vi "AutonSelector.vi"(10 "Buttons1":T1, 11 "Buttons in":T1) -> (0 "Current Auton":dbl, 1 "sorted array":string[](array[string]), 2 "Auton Array":dbl[][](array[numeric]), 3 "Number of Auton Files":dbl)   [LabVIEW 2013]
uses:
  <vilib>/Rock Robotics/WPI/Joystick/WPI_JoystickButtonState.ctl
  Robot Global Data.vi
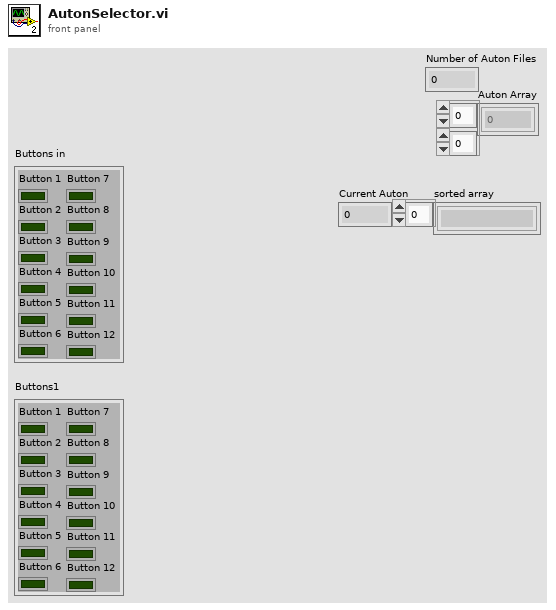
[diagram p1: front panel]
types:
  T1 = typedef "WPI_JoystickButtonState.ctl" = cluster{"Button 1":bool, "Button 2":bool, "Button 3":bool, "Button 4":bool, "Button 5":bool, "Button 6":bool, "Button 7":bool, "Button 8":bool, "Button 9":bool, "Button 10":bool, "Button 11":bool, "Button 12":bool}
  T2 = cluster{"Setpoint 1":dbl, "Setpoint 2":dbl, "Setpoint 3":dbl, "Setpoint 4":dbl, "RotLow":dbl, "RotHigh":dbl, "ExtLow":dbl, "ExtHigh":dbl}
  T3 = cluster{"FlipperLeftUp":dbl, "FlipperLeftDown":dbl, "FlipperRightUp":dbl, "FlipperRightDown":dbl, "KickerLeftBack":dbl, "KickerLeftForward":dbl, "KickerRightBack":dbl, "KickerRightForward":dbl}
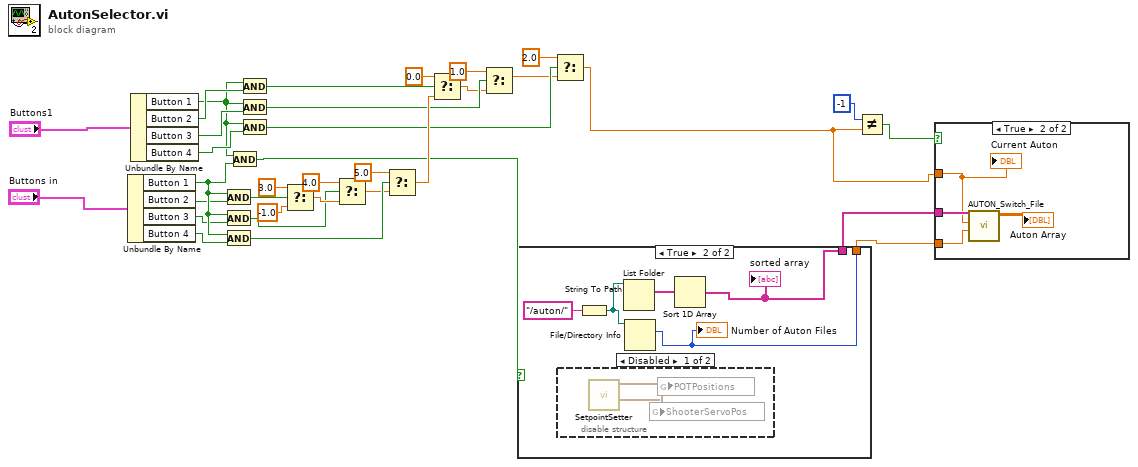
[diagram p0: block diagram]
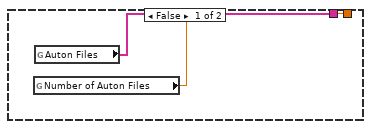
[diagram p3: hidden frame]
diagram:
  n1 = Unbundle By Name("Buttons in") -> ("Button 1"=w6:bool, "Button 2"=w4:bool, "Button 3"=w5:bool, "Button 4"=w7:bool)
  n2 = Unbundle By Name("Buttons1") -> ("Button 1"=w25:bool, "Button 2"=w26:bool, "Button 3"=w27:bool, "Button 4"=w28:bool)
  n3 = And(x=w6, y=w4) -> (x .and. y?=w8:bool)
  n4 = And(x=w6, y=w5) -> (x .and. y?=w11:bool)
  n5 = And(x=w6, y=w7) -> (x .and. y?=w17:bool)
  n6 = And(x=w25, y=w6) -> (x .and. y?=w15:bool)
  n7 = And(x=w25, y=w26) -> (x .and. y?=w24:bool)
  n8 = And(x=w25, y=w27) -> (x .and. y?=w22:bool)
  n9 = And(x=w25, y=w28) -> (x .and. y?=w29:bool)
  n10 = Select(t=3.0, s=w8, f=-1.0) -> (s? t:f=w12:dbl)
  n11 = Select(t=4.0, s=w11, f=w12) -> (s? t:f=w14:dbl)
  n12 = Select(t=5.0, s=w17, f=w14) -> (s? t:f=w30:dbl)
  n13 = Select(t=0.0, s=w24, f=w30) -> (s? t:f=w21:dbl)
  n14 = Select(t=1.0, s=w22, f=w21) -> (s? t:f=w19:dbl)
  n15 = case shown="True" w15 {
    tunnel: [w35 w37] -> w1
    tunnel: [w36 w38] -> w3
    frame False {
      n16 = global read "Robot Global Data.vi" "Number of Auton Files"() -> (w35:dbl)
      n17 = global read "Robot Global Data.vi" "Auton Files"() -> (w36:string[])
    }
    frame True {
      n18 = disable-structure shown="Disabled" {
        frame Disabled {
          n19 = call "SetpointSetter.vi"() -> ("Arm Pos"=w42:T2, "Shooter Servo Pos"=w43:T3)  [unwired: 10 in]
          n20 = global write "Robot Global Data.vi" "ShooterServoPos"(w43) -> ()
          n21 = global write "Robot Global Data.vi" "POTPositions"(w42) -> ()
        }
        frame Enabled {
        }
      }
      n22 = String To Path(string="/auton/") -> (path=w40:path)
      n23 = List Folder(path=w40) -> (filenames=w39:string[])  [unwired: 3 in, 3 out]
      n24 = File/Directory Info(path=w40) -> (size=w37:i64)  [unwired: 1 in, 6 out]
      "Number of Auton Files" <- w37
      n25 = Sort 1D Array(array=w39) -> (sorted array=w38:string[])
      "sorted array" <- w38
    }
  }
  n26 = Select(t=2.0, s=w29, f=w19) -> (s? t:f=w31:dbl)
  n27 = Not Equal?(x=-1, y=w31) -> (x != y?=w32:bool)
  n28 = case shown="True" w32 {
    tunnel: w3 -> [_ w47]
    tunnel: w1 -> [_ w46]
    tunnel: w31 -> [_ w45]
    frame False {
    }
    frame True {
      n29 = call "AUTON_Switch_File.vi"("Number of Auton Files"=w46, "Auton File"=w45, "Auton Files"=w47) -> ("Auton Array"=→"Auton Array":dbl[][])  [unwired: 7 in, 1 out]
      "Current Auton" <- w45
    }
  }
